vi "UpdateTest.vi"(8 "error in (no error)":errorcluster, 10 "Test":T1={"Code"="", "Name"="", "Description"="", "Group"="", "IsGroup"=FALSE, "Tag"="", "Method"="", "Parrameter"="", "DataType"=enum."String", "Value"=variant, "Status"=enum."Pass", "LimitLo"=variant, "LimitHi"=variant, "StringMatch"="", "BooleanMatch"=FALSE, "DisplayFormat"="", "Units"="", "TestTime"=0.0}, 11 "reference in":refnum<class "TestView_Tree_Single.lvclass">) -> (0 "error out":errorcluster, 3 "reference out":refnum<class "TestView_Tree_Single.lvclass">)   [LabVIEW 2022 SP3, in "TestView_Tree_Single.lvlib" / "TestView_Tree_Single.lvclass"]
uses:
  TestView_Tree_Single.lvclass
  Components/MES_Base.lvlibp/Controls/Test.ctl
  TestType.ctl
  <userlib>/_OpenG.lib/string/string.llb/Trim Whitespace (String Array)__ogtk.vi
  <userlib>/_OpenG.lib/string/string.llb/Trim Whitespace (String)__ogtk.vi
  Components/MES_Base.lvlibp/MES_Base.lvclass
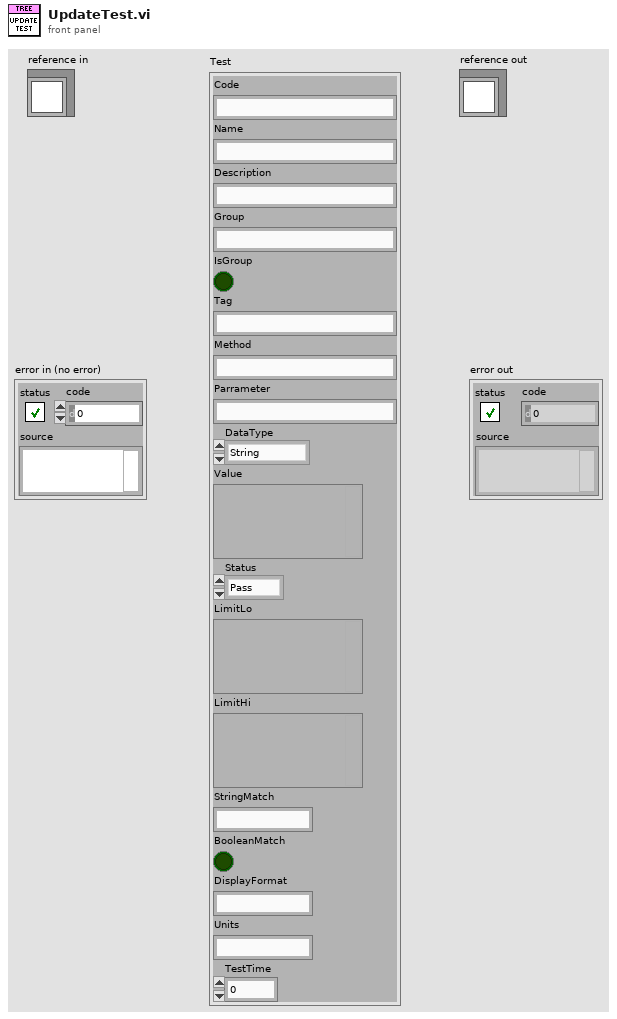
[diagram p1: front panel]
types:
  T1 = typedef "MES_Base.lvlibp/MES_Base.lvclass/Test.ctl" = cluster{"Code":string, "Name":string, "Description":string, "Group":string, "IsGroup":bool, "Tag":string, "Method":string, "Parrameter":string, "DataType":enum16{"NA", "String", "Boolean", "Int", "Dbl"}, "Value":variant, "Status":enum16{"Pending", "Pass", "Fail"}, "LimitLo":variant, "LimitHi":variant, "StringMatch":string, "BooleanMatch":bool, "DisplayFormat":string, "Units":string, "TestTime":dbl}
  T2 = typedef "TestView_Tree_Single.lvlib/TestView_Tree_Single.lvclass/TestType.ctl" = enum16{"null", "action", "action_active", "action_done", "group", "group_active", "group_fail", "group_pass", "test", "test_active", "test_fail", "test_pass", "warning"}
  T3 = typedef "TestView_Tree_Single.lvlib/TestView_Tree_Single.lvclass/ObjectAttributes.ctl" = cluster{"Front Panel":refnum<vi>, "Last_Item":string, "Config":T4, "Title":string, "User":string, "TreeRef":refnum<vi>, "Active DUT":i32, "Status":T5, "SN":string, "Spec":string}
  T4 = typedef "TestView_Tree_Single.lvlib/TestView_Tree_Single.lvclass/Config.ctl" = cluster{"default":string}
  T5 = typedef "TestView_Base.lvlibp/TestView_Base.lvclass/ViewStatus.ctl" = enum16{"Testing", "Ready", "Logout", "Login", "PASS", "FAIL", "FAULT", "ABORTED"}
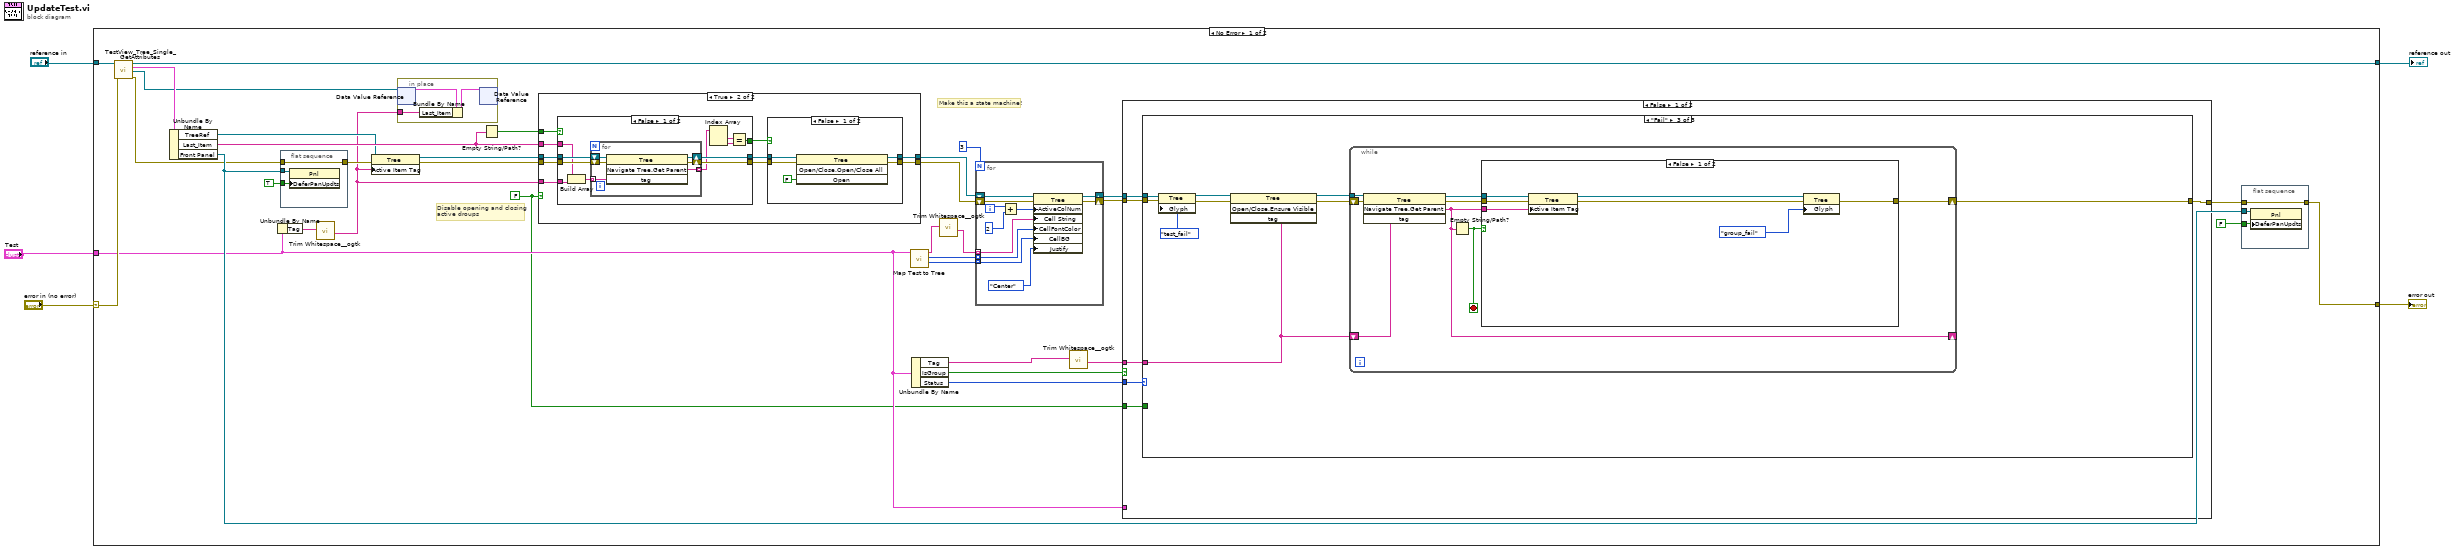
[diagram p0: block diagram]
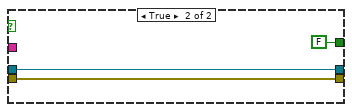
[diagram p3: hidden frame]
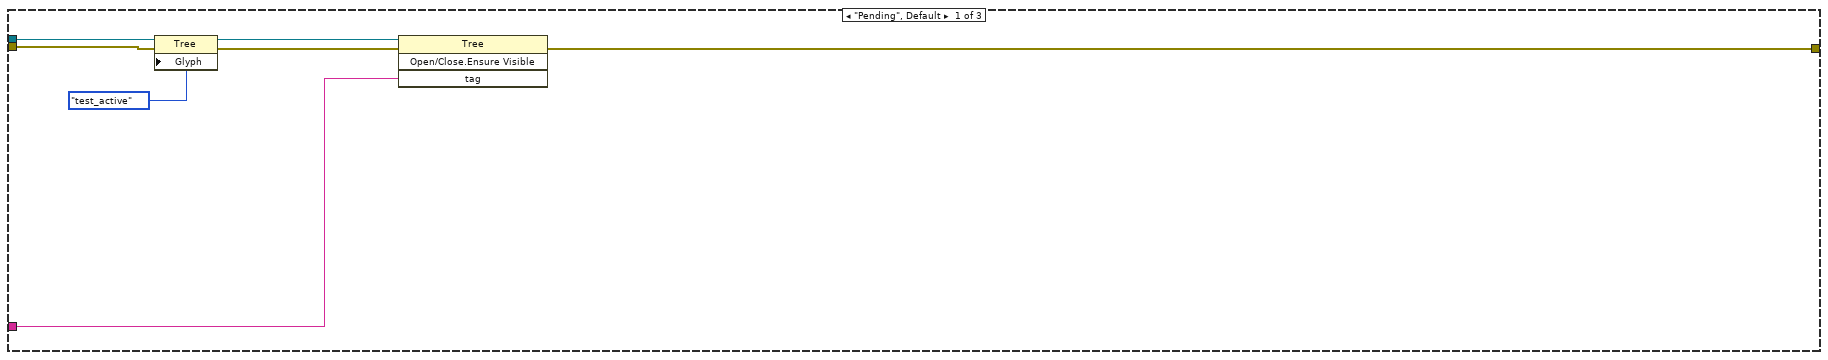
[diagram p5: hidden frame]
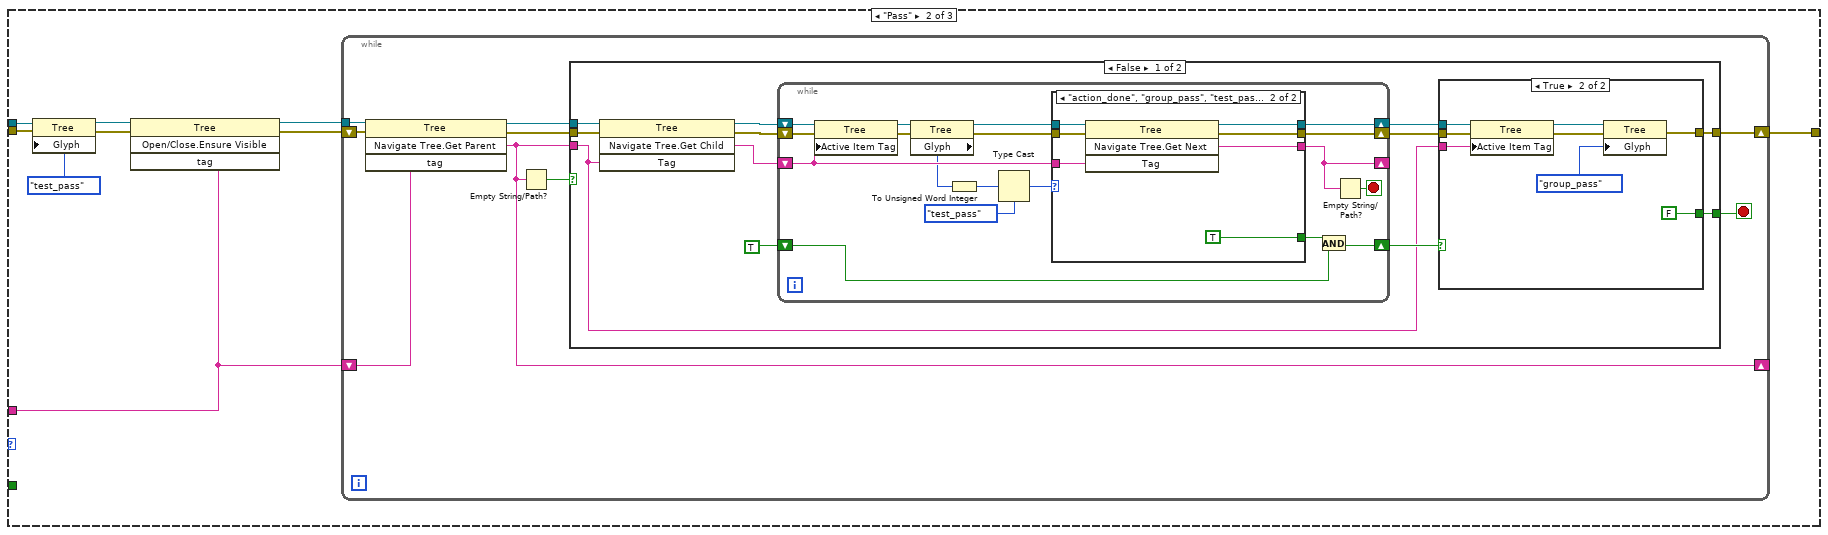
[diagram p6: hidden frame]
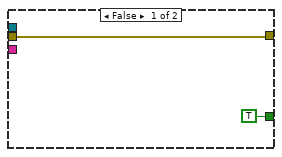
[diagram p7: hidden frame]
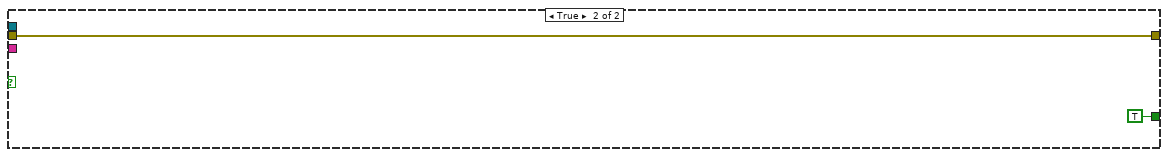
[diagram p9: hidden frame]
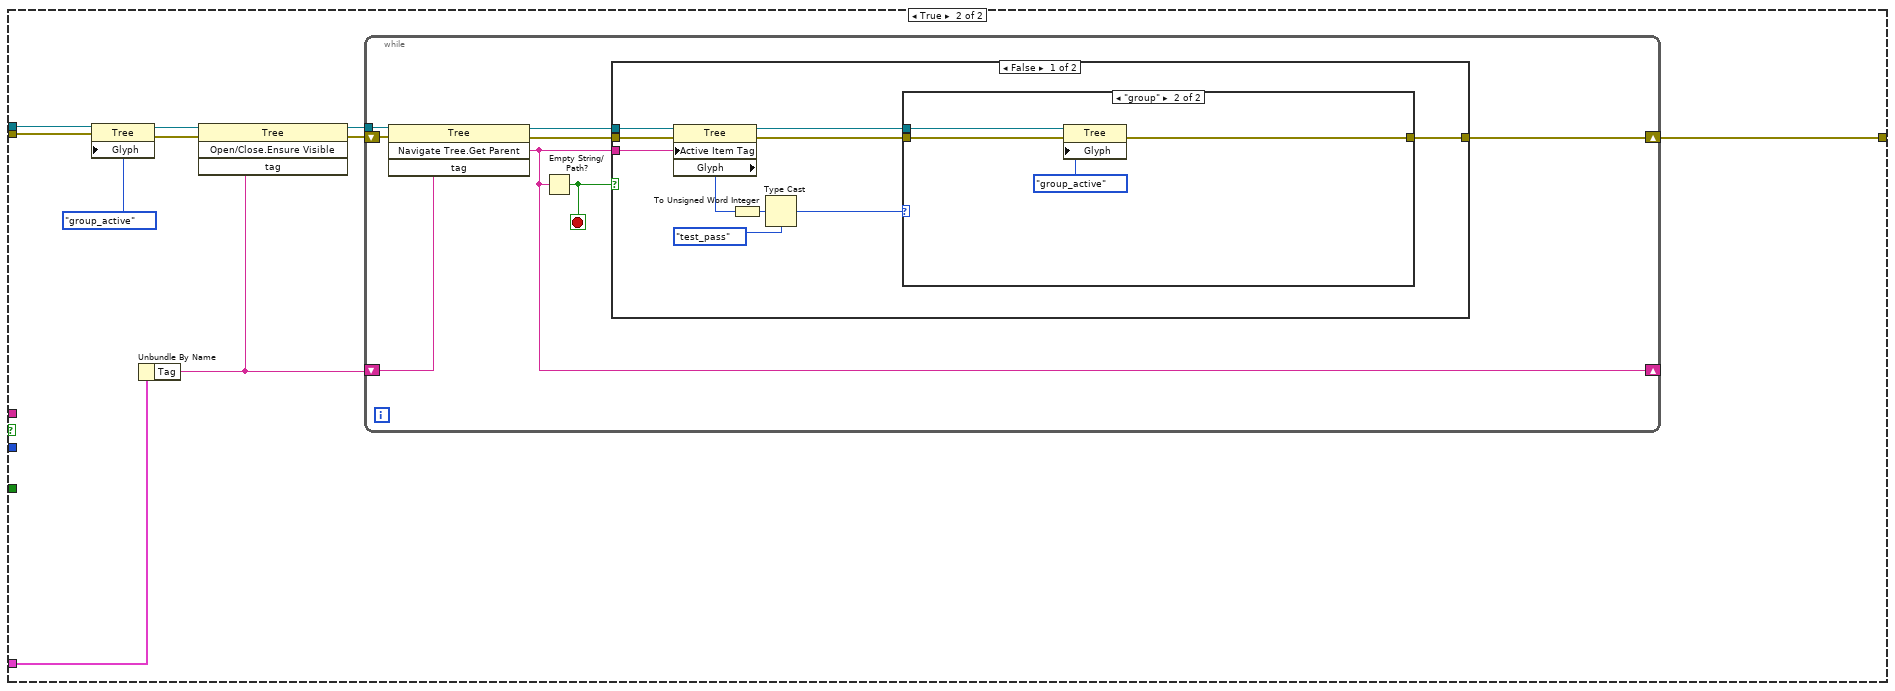
[diagram p11: hidden frame]
diagram:
  n1 = case shown="No Error" "error in (no error)" {
    selector: "error in (no error)" -> [w37 w241]
    tunnel: [w31 w241] -> w2
    tunnel: [w38 w240] -> w3
    tunnel: "reference in" -> [w39 w240]
    tunnel: "Test" -> [w18 _]
    frame No Error {
      w13 = FALSE
      # "Disable opening and closing\nactive droups"
      # "Make this a state machine!"
      n2 = call "TestView_Tree_Single_GetAttributes.vi"("error in (no error)"=w37, "reference in"=w39) -> ("error out"=w32:errorcluster, "DataRef"=w33:refnum<data-value>, "Data"=w36:T3, "reference out"=w38:refnum<class "TestView_Tree_Single.lvclass">)  [unwired: 6 in]
      n3 = Unbundle By Name(w36) -> ("TreeRef"=w16:refnum<vi>, "Last_Item"=w35:string, "Front Panel"=w34:refnum<vi>)
      n4 = Unbundle By Name(w18) -> ("Tag"=w8:string)
      n5 = flat-sequence {
        tunnel: w34 -> [w225]
        tunnel: TRUE ("Defer Panel Updates") -> [w224]
        tunnel: w32 -> [w223]
        tunnel: [w223] -> w17
        frame #0 {
          n6 = property class="Pnl"(reference=w225, "DeferPanUpdts"=w224) -> ()  [unwired: 1 in, 2 out]
        }
      }
      n7 = call-poly <userlib>:"Trim Whitespace__ogtk.vi"("String in"=w8) -> ("String out"=w7:string)  [unwired: 6 in]
      n8 = property class="Tree"(reference=w16, error in=w17, "Active Item Tag"=w7) -> (reference out=w15:refnum<vi>, error out=w14:errorcluster)
      n9 = in-place {
        in-place-border: w7 -> [w226]
        n10 = in-place-dvr #1(w33) -> (w228:T3)  [unwired: 1 out]
        n11 = Bundle By Name(cluster=w228, "Last_Item"=w226) -> (w227:T3)
        n12 = in-place-dvr #1(w227) -> ()  [unwired: 2 out]
      }
      n13 = Empty String/Path?(string/path=w35) -> (empty?=w28:bool)
      n14 = case shown="True" w13 {
        tunnel: w35 -> [_ w51]
        tunnel: [w40 w50] -> w29
        tunnel: w28 -> [_ w47]
        tunnel: [w41 w45] -> w25
        tunnel: w7 -> [_ w44]
        tunnel: w15 -> [w40 w43]
        tunnel: w14 -> [w41 w42]
        frame False {
        }
        frame True {
          n15 = case shown="False" w47 {
            tunnel: [w62 w71] -> w49
            tunnel: [w61 w70] -> w48
            tunnel: w42 -> [w59 w71]
            tunnel: w43 -> [w58 w70]
            tunnel: [w54 FALSE] -> w46
            tunnel: w44 -> [w53 _]
            tunnel: w51 -> [w52 _]
            frame False {
              n16 = Build Array(w52, w53) -> (w60:string[])
              n17 = for {
                tunnel: w60 -> [w64] mode=indexing
                shift-right: [w68] -> w62
                shift-left: w59 -> [w65]
                shift-right: [w67] -> w61
                shift-left: w58 -> [w66]
                tunnel: [w63] -> w57 mode=indexing
                n18 = invoke class="Tree" method="Navigate Tree.Get Parent"(reference=w66, error in=w65, "tag"=w64) -> (reference out=w67:refnum<vi>, error out=w68:errorcluster, "Navigate Tree:Get Parent"=w63:string)  [unwired: 1 in, 1 out]
              }
              n19 = Index Array(array=w57) -> (element #1=w56:string, element #2=w55:string)  [unwired: 2 in]
              n20 = Equal?(x=w56, y=w55) -> (x = y?=w54:bool)
            }
            frame True {
            }
          }
          n21 = case shown="False" w46 {
            tunnel: [w76 w78] -> w50
            tunnel: w49 -> [w75 w77]
            tunnel: [w73 w77] -> w45
            tunnel: w48 -> [w72 w78]
            frame False {
              n22 = invoke class="Tree" method="Open/Close.Open/Close All"(reference=w72, error in=w75, "Open"=FALSE ("Open?")) -> (reference out=w76:refnum<vi>, error out=w73:errorcluster)  [unwired: 1 in, 2 out]
            }
            frame True {
            }
          }
        }
      }
      n23 = call "Map Test to Tree.vi"("Test"=w18) -> ("BG Colour"=w19:u32[], "Text Colour"=w20:u32[], "Text"=w12:string[])  [unwired: 7 in, 1 out]
      n24 = Unbundle By Name(w18) -> ("Tag"=w10:string, "IsGroup"=w6:bool, "Status"=w21:enum16{"Pending", "Pass", "Fail"})
      n25 = call-poly <userlib>:"Trim Whitespace__ogtk.vi"("String in"=w12) -> ("String out"=w11:string[])  [unwired: 6 in]
      n26 = for {
        N: 3 -> [_]
        shift-right: [w238] -> w23
        shift-left: w29 -> [w239]
        shift-right: [w236] -> w24
        shift-left: w25 -> [w237]
        tunnel: w20 -> [w232] mode=indexing
        tunnel: w11 -> [w233] mode=indexing
        tunnel: w19 -> [w234] mode=indexing
        i -> [w231]
        n27 = Add(x=w231, y=2) -> (x+y=w229:i32)
        n28 = property class="Tree"(reference=w239, error in=w237, "ActiveColNum"=w229, "Cell String"=w233, "CellFontColor"=w232, "CellBG"=w234, "Justify"=enum16{"Left", "Center", "Right"}."Center" ("Active Cell:Cell Justification")) -> (reference out=w238:refnum<vi>, error out=w236:errorcluster)
      }
      n29 = call-poly <userlib>:"Trim Whitespace__ogtk.vi"("String in"=w10) -> ("String out"=w9:string)  [unwired: 6 in]
      n30 = case shown="False" w6 {
        tunnel: w24 -> [w83 w189]
        tunnel: w23 -> [w84 w190]
        tunnel: w18 -> [_ w188]
        tunnel: [w81 w187] -> w22
        tunnel: w9 -> [w82 _]
        tunnel: w21 -> [w80 _]
        tunnel: w13 -> [w79 _]
        frame False {
          n31 = case shown="\"Fail\"" w80 {
            tunnel: w84 -> [w89 w100 w169]
            tunnel: w83 -> [w88 w99 w168]
            tunnel: w82 -> [w86 w98 w167]
            tunnel: [w87 w97 w166] -> w81
            tunnel: w79 -> [_ _ _]
            frame "Pending", Default {
              n32 = property class="Tree"(reference=w89, error in=w88, "Glyph"=TestType."test_active" ("glyph")) -> (reference out=w90:refnum<vi>, error out=w91:errorcluster)
              n33 = invoke class="Tree" method="Open/Close.Ensure Visible"(reference=w90, error in=w91, "tag"=w86) -> (error out=w87:errorcluster)  [unwired: 1 in, 3 out]
            }
            frame "Pass" {
              n34 = property class="Tree"(reference=w100, error in=w99, "Glyph"=TestType."test_pass" ("glyph")) -> (reference out=w95:refnum<vi>, error out=w96:errorcluster)
              n35 = invoke class="Tree" method="Open/Close.Ensure Visible"(reference=w95, error in=w96, "tag"=w98) -> (reference out=w94:refnum<vi>, error out=w93:errorcluster)  [unwired: 1 in, 2 out]
              n36 = while {
                tunnel: w94 -> [w109]
                shift-right: [w104] -> _
                shift-left: w98 -> [w107]
                shift-right: [w102] -> w97
                shift-left: w93 -> [w108]
                stop <- w101 stop-if-true
                n37 = invoke class="Tree" method="Navigate Tree.Get Parent"(reference=w109, error in=w108, "tag"=w107) -> (reference out=w106:refnum<vi>, error out=w105:errorcluster, "Navigate Tree:Get Parent"=w104:string)  [unwired: 1 in, 1 out]
                n38 = Empty String/Path?(string/path=w104) -> (empty?=w103:bool)
                n39 = case shown="False" w103 {
                  tunnel: w106 -> [w115 _]
                  tunnel: w105 -> [w114 w160]
                  tunnel: w104 -> [w111 _]
                  tunnel: [w121 w160] -> w102
                  tunnel: [w110 TRUE] -> w101
                  frame False {
                    n40 = invoke class="Tree" method="Navigate Tree.Get Child"(reference=w115, error in=w114, "Tag"=w111) -> (reference out=w120:refnum<vi>, error out=w119:errorcluster, "Navigate Tree:Get Child"=w116:string)  [unwired: 1 in, 1 out]
                    n41 = while {
                      shift-right: [w148] -> w118
                      shift-left: w120 -> [w143]
                      shift-right: [w149] -> w117
                      shift-left: w119 -> [w141]
                      shift-right: [w147] -> _
                      shift-left: w116 -> [w139]
                      shift-right: [w135] -> w112
                      shift-left: TRUE -> [w134]
                      stop <- w146 stop-if-true
                      n42 = property class="Tree"(reference=w143, error in=w141, "Active Item Tag"=w139) -> (reference out=w142:refnum<vi>, error out=w140:errorcluster)
                      n43 = property class="Tree"(reference=w142, error in=w140) -> (reference out=w145:refnum<vi>, error out=w144:errorcluster, "Glyph"=w138:i32)
                      n44 = To Unsigned Word Integer(number=w138) -> (unsigned 16bit integer=w133:u16)
                      n45 = Type Cast(type=TestType."test_pass" ("glyph"), x=w133) -> (*(type *) &x=w137:T2)
                      n46 = case shown="\"action_done\", \"group_pass\", \"test_pass\"" w137 {
                        tunnel: [w150 w158] -> w149
                        tunnel: [w151 w157] -> w148
                        tunnel: [_ w156] -> w147
                        tunnel: w145 -> [w151 w155]
                        tunnel: w144 -> [w150 w154]
                        tunnel: w139 -> [_ w153]
                        tunnel: [_ TRUE] -> w136
                        frame "null", Default {
                        }
                        frame "action_done", "group_pass", "test_pass" {
                          n47 = invoke class="Tree" method="Navigate Tree.Get Next"(reference=w155, error in=w154, "Tag"=w153) -> (reference out=w157:refnum<vi>, error out=w158:errorcluster, "Navigate Tree:Get Next Item"=w156:string)  [unwired: 1 in, 1 out]
                        }
                      }
                      n48 = And(x=w136, y=w134) -> (x .and. y?=w135:bool)
                      n49 = Empty String/Path?(string/path=w147) -> (empty?=w146:bool)
                    }
                    n50 = case shown="True" w112 {
                      tunnel: [w123 w131] -> w121
                      tunnel: w118 -> [_ w130]
                      tunnel: w117 -> [w123 w128]
                      tunnel: w111 -> [_ w126]
                      tunnel: [TRUE FALSE] -> w110
                      frame False {
                      }
                      frame True {
                        n51 = property class="Tree"(reference=w130, error in=w128, "Active Item Tag"=w126) -> (reference out=w129:refnum<vi>, error out=w127:errorcluster)
                        n52 = property class="Tree"(reference=w129, error in=w127, "Glyph"=TestType."group_pass" ("glyph")) -> (error out=w131:errorcluster)  [unwired: 1 out]
                      }
                    }
                  }
                  frame True {
                  }
                }
              }
            }
            frame "Fail" {
              n53 = property class="Tree"(reference=w169, error in=w168, "Glyph"=TestType."test_fail" ("glyph")) -> (reference out=w164:refnum<vi>, error out=w165:errorcluster)
              n54 = invoke class="Tree" method="Open/Close.Ensure Visible"(reference=w164, error in=w165, "tag"=w167) -> (reference out=w163:refnum<vi>, error out=w162:errorcluster)  [unwired: 1 in, 2 out]
              n55 = while {
                tunnel: w163 -> [w177]
                shift-right: [w172] -> _
                shift-left: w167 -> [w175]
                shift-right: [w170] -> w166
                shift-left: w162 -> [w176]
                stop <- w171 stop-if-true
                n56 = invoke class="Tree" method="Navigate Tree.Get Parent"(reference=w177, error in=w176, "tag"=w175) -> (reference out=w174:refnum<vi>, error out=w173:errorcluster, "Navigate Tree:Get Parent"=w172:string)  [unwired: 1 in, 1 out]
                n57 = Empty String/Path?(string/path=w172) -> (empty?=w171:bool)
                n58 = case shown="False" w171 {
                  tunnel: w174 -> [w184 _]
                  tunnel: w173 -> [w183 w185]
                  tunnel: w172 -> [w182 _]
                  tunnel: [w179 w185] -> w170
                  frame False {
                    n59 = property class="Tree"(reference=w184, error in=w183, "Active Item Tag"=w182) -> (reference out=w181:refnum<vi>, error out=w180:errorcluster)
                    n60 = property class="Tree"(reference=w181, error in=w180, "Glyph"=TestType."group_fail" ("glyph")) -> (error out=w179:errorcluster)  [unwired: 1 out]
                  }
                  frame True {
                  }
                }
              }
            }
          }
        }
        frame True {
          n61 = property class="Tree"(reference=w190, error in=w189, "Glyph"=TestType."group_active" ("glyph")) -> (reference out=w192:refnum<vi>, error out=w191:errorcluster)
          n62 = Unbundle By Name(w188) -> ("Tag"=w195:string)
          n63 = invoke class="Tree" method="Open/Close.Ensure Visible"(reference=w192, error in=w191, "tag"=w195) -> (reference out=w193:refnum<vi>, error out=w194:errorcluster)  [unwired: 1 in, 2 out]
          n64 = while {
            tunnel: w193 -> [w203]
            shift-right: [w198] -> _
            shift-left: w195 -> [w201]
            shift-right: [w196] -> w187
            shift-left: w194 -> [w202]
            stop <- w197 stop-if-true
            n65 = invoke class="Tree" method="Navigate Tree.Get Parent"(reference=w203, error in=w202, "tag"=w201) -> (reference out=w200:refnum<vi>, error out=w199:errorcluster, "Navigate Tree:Get Parent"=w198:string)  [unwired: 1 in, 1 out]
            n66 = Empty String/Path?(string/path=w198) -> (empty?=w197:bool)
            n67 = case shown="False" w197 {
              tunnel: w200 -> [w213 _]
              tunnel: w199 -> [w212 w219]
              tunnel: w198 -> [w211 _]
              tunnel: [w208 w219] -> w196
              frame False {
                n68 = property class="Tree"(reference=w213, error in=w212, "Active Item Tag"=w211) -> (reference out=w210:refnum<vi>, error out=w209:errorcluster, "Glyph"=w206:i32)
                n69 = To Unsigned Word Integer(number=w206) -> (unsigned 16bit integer=w207:u16)
                n70 = Type Cast(type=TestType."test_pass" ("glyph"), x=w207) -> (*(type *) &x=w205:T2)
                n71 = case shown="\"group\"" w205 {
                  tunnel: w210 -> [_ w218]
                  tunnel: w209 -> [w214 w217]
                  tunnel: [w214 w216] -> w208
                  frame "null", Default {
                  }
                  frame "group" {
                    n72 = property class="Tree"(reference=w218, error in=w217, "Glyph"=TestType."group_active" ("glyph")) -> (error out=w216:errorcluster)  [unwired: 1 out]
                  }
                }
              }
              frame True {
              }
            }
          }
        }
      }
      n73 = flat-sequence {
        tunnel: w34 -> [w222]
        tunnel: FALSE ("Defer Panel Updates") -> [w221]
        tunnel: w22 -> [w220]
        tunnel: [w220] -> w31
        frame #0 {
          n74 = property class="Pnl"(reference=w222, "DeferPanUpdts"=w221) -> ()  [unwired: 1 in, 2 out]
        }
      }
    }
    frame Error {
    }
  }
  "error out" <- w2
  "reference out" <- w3
